vi "Constant - Queue Name.vi"() -> (0 "Queue Name":string)   [LabVIEW 2022 SP3]
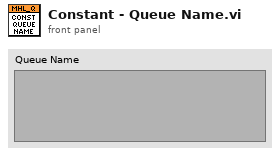
[diagram p1: front panel]
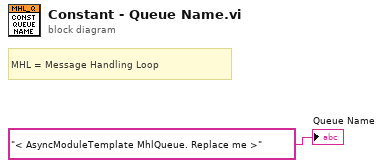
[diagram p0: block diagram]
diagram:
  # "MHL = Message Handling Loop"
  "Queue Name" <- "< AsyncModuleTemplate MhlQueue. Replace me >" ("Queue Name")
